vi "Set Screw Printing Speed.vi"(8 "error in (no error)":errorcluster, 10 "Print Speed":u16(ring)=1 items=["0%"=1, "25%"=225, "50%"=450, "75%"=675, "100%"=900], 11 "Feeder Actor.lvlib:Screw.lvclass":refnum<class "Screw.lvclass">) -> (0 "error out":errorcluster, 3 "Feeder Actor.lvlib:Screw.lvclass 2":refnum<class "Screw.lvclass">)   [LabVIEW 2018, in "Feeder Actor.lvlib" / "Screw.lvclass"]
uses:
  Screw.lvclass
  Screw.lvclass/Screw.ctl
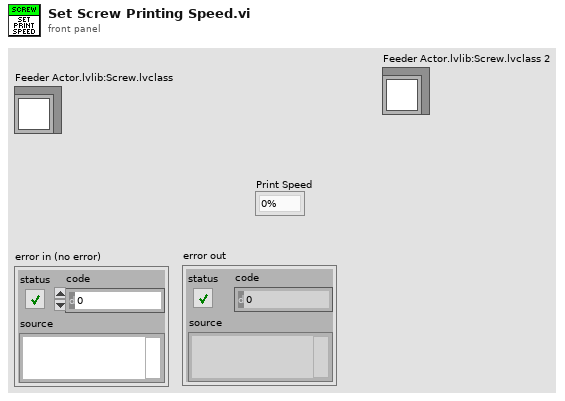
[diagram p1: front panel]
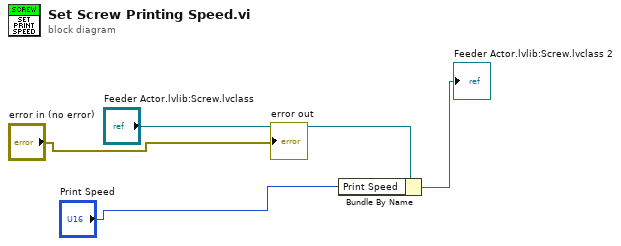
[diagram p0: block diagram]
diagram:
  n1 = Bundle By Name(cluster="Feeder Actor.lvlib:Screw.lvclass", "Print Speed"="Print Speed") -> (→"Feeder Actor.lvlib:Screw.lvclass 2":refnum<class "Screw.lvclass">)
  "error out" <- "error in (no error)"
